vi "Read Gas Correction Configuration.vi"(8 "error in (no error)":errorcluster, 11 "VGC in":refnum<class "PL Inficon VGC.lvclass">) -> (0 "error out":errorcluster, 2 "gas correction":u16[](array[ring]) items=["nitrogen/air", "argon", "hydrogen", "helium", "neon", "krypton", "xenon", "other"], 3 "VGC out":refnum<class "PL Inficon VGC.lvclass">)   [LabVIEW 2015, in "PL Inficon VGC.lvclass"]
doc: "Reads gas type correction configuration."
uses:
  PL Inficon VGC.lvclass
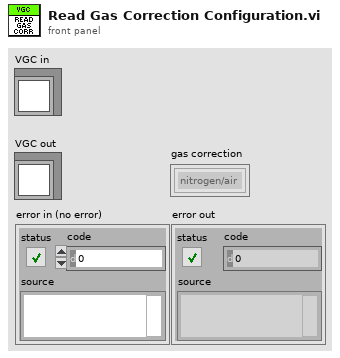
[diagram p1: front panel]
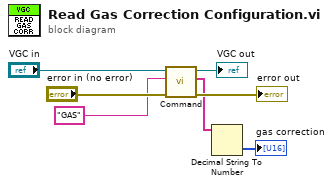
[diagram p0: block diagram]
diagram:
  n1 = call "Command.vi"("error in (no error)"="error in (no error)", "command"="GAS" ("format string"), "VGC in"="VGC in") -> ("error out"=→"error out":errorcluster, "response data"=w3:string[], "VGC out"=→"VGC out":refnum<class "PL Inficon VGC.lvclass">)  [unwired: 6 in]
  n2 = Decimal String To Number(string=w3) -> (number=→"gas correction":i32[])  [unwired: 2 in, 1 out]
